vi "write_spreadsheet.vi"() -> ()   [LabVIEW 2021]
uses:
  <vilib>/Utility/file.llb/Write Delimited Spreadsheet (DBL).vi
panel:
  out "file path":path
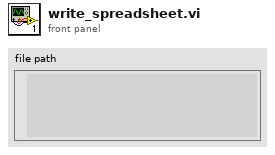
[diagram p1: front panel]
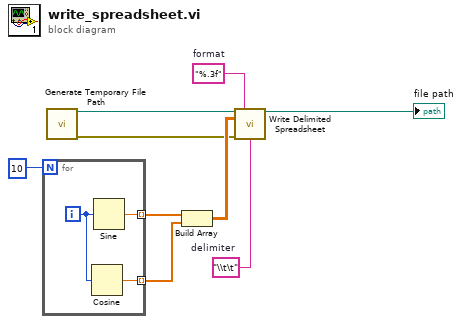
[diagram p0: block diagram]
diagram:
  w1 = "\\t\t"  # delimiter
  w5 = "%.3f"  # format
  n1 = for {
    N: 10 -> [_]
    tunnel: [w11] -> w8 mode=indexing
    tunnel: [w10] -> w7 mode=indexing
    i -> [w12]
    n2 = Cosine(x=w12) -> (cos(x)=w10:dbl)
    n3 = Sine(x=w12) -> (sin(x)=w11:dbl)
  }
  n4 = call <vilib>:"Generate Temporary File Path.vi"() -> ("error out"=w3:errorcluster, "Unique Temporary File Path"=w4:path)  [unwired: 10 in]
  n5 = Build Array(w8, w7) -> (w6:dbl[][])
  n6 = call-poly <vilib>:"Write Delimited Spreadsheet.vi"("file path (dialog if empty)"=w4, "format (%.3f)"=w5, "2D data"=w6, "error in (no error)"=w3, "delimiter (\\t)"=w1) -> ("new file path (Not A Path if cancelled)"=→"file path":path)  [unwired: 9 in, 1 out]
